vi "Begin.vi"(8 "error in":errorcluster) -> (0 "error out":errorcluster)   [LabVIEW 2014]
doc: "Called before other user functions, this VI is expected to open initial I/O refnums, load in file data, and do all program initialization. Notice that the <B>error out</B> terminal is simply used for data flow. Wiring it to other structures or subVIs ensures that this VI runs first."
uses:
  <vilib>/Rock Robotics/WPI/DriverStation/WPI_DriverStationRobotMode2.ctl
  <vilib>/Rock Robotics/WPI/Joystick/WPI_JoystickDeviceEnum.ctl
  <vilib>/Rock Robotics/SystemInterfaces/DIO/FPGA_DIOChannel.ctl
  <vilib>/Rock Robotics/SystemInterfaces/AI/FPGA_AIChannel.ctl
  <vilib>/Rock Robotics/SystemInterfaces/Typedef/FPGA_TypedefAnalogModule.ctl
  <vilib>/Rock Robotics/SystemInterfaces/DIO/FPGA_DIORelayChannel.ctl
  <vilib>/Rock Robotics/SystemInterfaces/DIO/FPGA_DIOPWMChannel.ctl
  <vilib>/Rock Robotics/SystemInterfaces/Typedef/FPGA_TypedefDigitalModule.ctl
  Robot Global Data.vi
  <vilib>/Rock Robotics/Network Tables/SD Write String Array.vi
  <vilib>/Rock Robotics/WPI/Counter/WPI_CounterDigitalInputToDigitalSource.vi
  <vilib>/Rock Robotics/WPI/MotorControl/WPI_MotorControlOpen Talon.vi
  <vilib>/Rock Robotics/WPI/Compressor/WPI_CompressorGetSetRefNum.vi
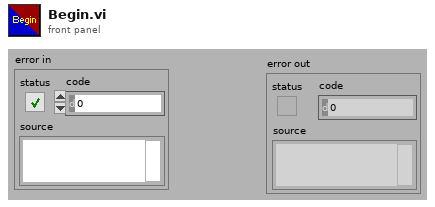
[diagram p1: front panel]
types:
  T1 = typedef "FPGA_TypedefDigitalModule.ctl" = enum16{"Controller 1"}
  T2 = typedef "FPGA_DIOPWMChannel.ctl" = enum8{"PWM 0", "PWM 1", "PWM 2", "PWM 3", "PWM 4", "PWM 5", "PWM 6", "PWM 7", "PWM 8", "PWM 9", "PWM MXP 0", "PWM MXP 1", "PWM MXP 2", "PWM MXP 3", "PWM MXP 4", "PWM MXP 5", "PWM MXP 6", "PWM MXP 7", "PWM MXP 8", "PWM MXP 9", "Invalid"}
  T3 = typedef "FPGA_DIOChannel.ctl" = enum8{"DIO 0", "DIO 1", "DIO 2", "DIO 3", "DIO 4", "DIO 5", "DIO 6", "DIO 7", "DIO 8", "DIO 9", "DIO MXP 0", "DIO MXP 1", "DIO MXP 2", "DIO MXP 3", "DIO MXP 4", "DIO MXP 5", "DIO MXP 6", "DIO MXP 7", "DIO MXP 8", "DIO MXP 9", "DIO MXP 10", "DIO MXP 11", "DIO MXP 12", "DIO MXP 13", "DIO MXP 14", "DIO MXP 15", "Invalid"}
  T4 = typedef "FPGA_DIORelayChannel.ctl" = enum8{"Relay 0", "Relay 1", "Relay 2", "Relay 3", "Invalid"}
  T5 = typedef "FPGA_TypedefAnalogModule.ctl" = enum16{"Controller 1"}
  T6 = typedef "FPGA_AIChannel.ctl" = enum8{"AI 0", "AI 1", "AI 2", "AI 3", "AI MXP 0", "AI MXP 1", "AI MXP 2", "AI MXP 3", "Invalid"}
  T7 = typedef "WPI_JoystickDeviceEnum.ctl" = enum16{"USB 0", "USB 1", "USB 2", "USB 3", "USB 4", "USB 5"}
  T8 = typedef "WPI_DriverStationRobotMode2.ctl" = enum16{"Autonomous Disabled", "Autonomous Enabled", "Teleop Disabled", "Teleop Enabled", "Disconnected", "Finish", "Test Disabled", "Test Enabled", "Emergency Stopped"}
  T9 = typedef "WPI_MotorControlDeviceRef.ctl" = cluster{"DeviceStatus":errorcluster, "Type":T10, "PWM":cluster{"Controller":T1, "PWM Channel":T2, "DeadBand":T11}, "CAN":cluster{"Device Number":u8, "Control Mode":T12, "Semaphore":T13, "Max Vout":dbl, "TalonSRX Control Mode":T14}, "Invert":bool, "TransformRef":T15, "InvTransformRef":T15}
  T10 = typedef "WPI_MotorControlType.ctl" = enum16{"PWM", "CAN", "CANTalonSRX"}
  T11 = typedef "WPI_PWMDeadband.ctl" = cluster{"Name":string, "maxPositivePwm":i32, "minPositivePwm":i32, "centerPwm":i32, "maxNegativePwm":i32, "minNegativePwm":i32, "angularRange":u16}
  T12 = typedef "WPI_CANJaguar_ControlMode.ctl" = enum8{"Percent VBus", "Current", "Speed", "Position", "Voltage"}
  T13 = typedef "Semaphore RefNum" = refnum<k1>
  T14 = typedef "WPI_CANTalonSRX_APIControlMode.ctl" = enum8{"Percent VBus", "Speed", "Position", "Slave", "Unchanged / Invalid"}
  T15 = typedef "WPI_PWMTransform_ConPane.ctl" = refnum<vi>
  T16 = typedef "WPI_DigitalInputDevRef.ctl" = cluster{"DevStatus":errorcluster, "DIO Channel":T3, "Controller":T1}
  T17 = typedef "FPGA_CounterEncoderSourceConvertionLVSourceType.ctl" = cluster{"DevStatus":errorcluster, "AnalogTriggerMode?":bool, "DigitalMode":cluster{"Controller":T1, "DIO Channel":T18}, "AnalogTriggerMode":cluster{"AnalogTriggerIndex":T19, "OutputType":T20}}
  T18 = typedef "FPGA_DIODigitalSourceChannel.ctl" = enum8{"DIO 0", "DIO 1", "DIO 2", "DIO 3", "DIO 4", "DIO 5", "DIO 6", "DIO 7", "DIO 8", "DIO 9", "DIO MXP 0", "DIO MXP 1", "DIO MXP 2", "DIO MXP 3", "DIO MXP 4", "DIO MXP 5", "DIO MXP 6", "DIO MXP 7", "DIO MXP 8", "DIO MXP 9", "DIO MXP 10", "DIO MXP 11", "DIO MXP 12", "DIO MXP 13", "DIO MXP 14", "DIO MXP 15", "Disabled"}
  T19 = typedef "FPGA_AnalogTriggerIndex.ctl" = enum8{"Trig 0", "Trig 1", "Trig 2", "Trig 3", "Trig 4", "Trig 5", "Trig 6", "Trig 7", "Invalid"}
  T20 = typedef "FPGA_AnalogTriggerOutType.ctl" = enum16{"InWindow", "TriggerState", "Rising", "Falling"}
  T21 = typedef "WPI_EncoderDevRef.ctl" = cluster{"DevStatus":errorcluster, "EncoderIndex":T22, "CounterIndex":T23, "DistancePerCount":dbl, "Decoding Type":T24}
  T22 = typedef "FPGA_EncoderIdx.ctl" = enum8{"Enc 0", "Enc 1", "Enc 2", "Enc 3", "Enc 4", "Enc 5", "Enc 6", "Enc 7", "Invalid"}
  T23 = typedef "FPGA_CounterCtrSystemIndex.ctl" = enum8{"Ctr 0", "Ctr 1", "Ctr 2", "Ctr 3", "Ctr 4", "Ctr 5", "Ctr 6", "Ctr 7", "Invalid"}
  T24 = typedef "WPI_EncoderType.ctl" = enum16{"1x", "2x", "4x"}
  T25 = typedef "WPI_RelayDevRef.ctl" = cluster{"DevStatus":errorcluster, "Relay Channel":T4, "Controller":T1, "Relay Direction":T26}
  T26 = typedef "WPI_RelayDirection.ctl" = enum16{"Both directions", "Forward only", "Reverse only"}
  T27 = typedef "WPI_CompressorDevRef.ctl" = cluster{"DevStatus":errorcluster, "Pneumatics Control Module":u8}
  T28 = typedef "WPI_JoystickDevRef.ctl" = cluster{"Device":T7}
  T29 = typedef "WPI_AnalogChannelDevRef.ctl" = cluster{"DevStatus":errorcluster, "Controller":T5, "Analog Channel":T6}
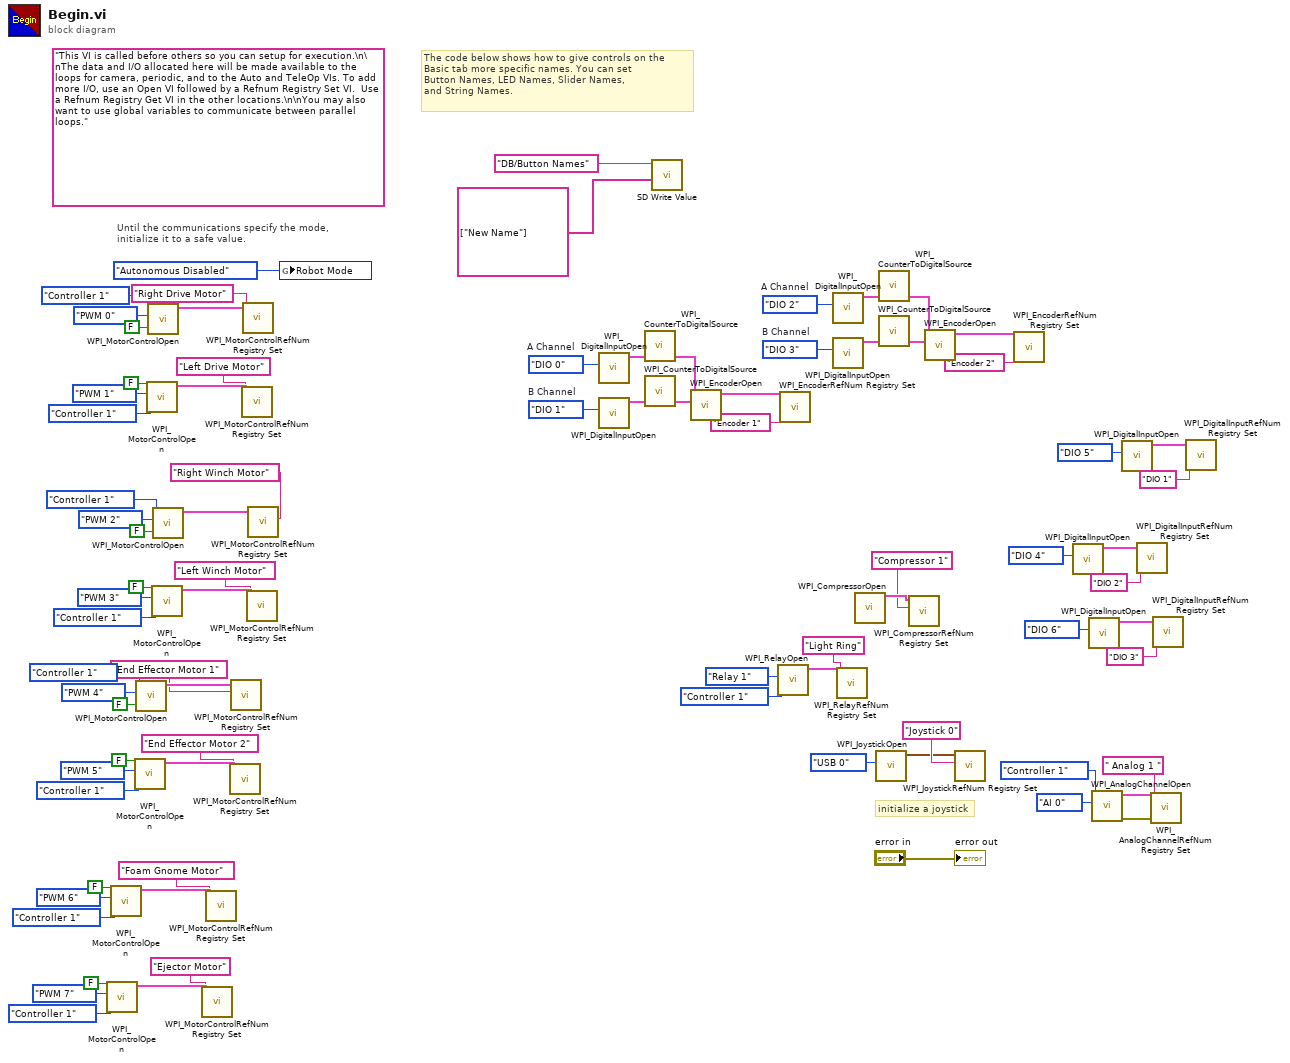
[diagram p0: block diagram]
diagram:
  w65 = FPGA_DIOChannel."DIO 3"  # B Channel
  w64 = FPGA_DIOChannel."DIO 2"  # A Channel
  w76 = FPGA_DIOChannel."DIO 1"  # B Channel
  w75 = FPGA_DIOChannel."DIO 0"  # A Channel
  (unwired) "This VI is called before others so you can setup for execution.\n\nThe data and I/O allocated here will be made available to the loops for camera, periodic, and to the Auto and TeleOp VIs. To add more I/O, use an Open VI followed by a Refnum Registry Set VI.  Use a Refnum Registry Get VI in the other locations.\n\nYou may also want to use global variables to communicate between parallel loops."
  # "The code below shows how to give controls on the\nBasic tab more specific names. You can set\nButton Names, LED Names, Slider Names,\nand String Names."
  # "initialize a joystick"
  # "Until the communications specify the mode,\ninitialize it to a safe value."
  n1 = call-poly <vilib>:"WPI_MotorControlOpen.vi"("Eliminate Deadband"=FALSE, "PWM Channel"=FPGA_DIOPWMChannel."PWM 7", "Controller"=FPGA_TypedefDigitalModule."Controller 1") -> ("MotorControlDeviceRef"=w7:T9)  [unwired: 7 in, 1 out]
  n2 = call-poly <vilib>:"WPI_MotorControlOpen.vi"("Eliminate Deadband"=FALSE, "PWM Channel"=FPGA_DIOPWMChannel."PWM 6", "Controller"=FPGA_TypedefDigitalModule."Controller 1") -> ("MotorControlDeviceRef"=w12:T9)  [unwired: 7 in, 1 out]
  n3 = call-poly <vilib>:"WPI_MotorControlOpen.vi"("Eliminate Deadband"=FALSE, "PWM Channel"=FPGA_DIOPWMChannel."PWM 5", "Controller"=FPGA_TypedefDigitalModule."Controller 1") -> ("MotorControlDeviceRef"=w20:T9)  [unwired: 7 in, 1 out]
  n4 = call-poly <vilib>:"WPI_MotorControlOpen.vi"("Eliminate Deadband"=FALSE, "PWM Channel"=FPGA_DIOPWMChannel."PWM 4", "Controller"=FPGA_TypedefDigitalModule."Controller 1") -> ("MotorControlDeviceRef"=w21:T9)  [unwired: 7 in, 1 out]
  n5 = call-poly <vilib>:"WPI_MotorControlOpen.vi"("Eliminate Deadband"=FALSE, "PWM Channel"=FPGA_DIOPWMChannel."PWM 1", "Controller"=FPGA_TypedefDigitalModule."Controller 1") -> ("MotorControlDeviceRef"=w39:T9)  [unwired: 7 in, 1 out]
  n6 = call-poly <vilib>:"WPI_MotorControlOpen.vi"("Eliminate Deadband"=FALSE, "PWM Channel"=FPGA_DIOPWMChannel."PWM 0", "Controller"=FPGA_TypedefDigitalModule."Controller 1") -> ("MotorControlDeviceRef"=w40:T9)  [unwired: 7 in, 1 out]
  n7 = call-poly <vilib>:"WPI_MotorControlOpen.vi"("Eliminate Deadband"=FALSE, "PWM Channel"=FPGA_DIOPWMChannel."PWM 3", "Controller"=FPGA_TypedefDigitalModule."Controller 1") -> ("MotorControlDeviceRef"=w29:T9)  [unwired: 7 in, 1 out]
  n8 = call-poly <vilib>:"WPI_MotorControlOpen.vi"("Eliminate Deadband"=FALSE, "PWM Channel"=FPGA_DIOPWMChannel."PWM 2", "Controller"=FPGA_TypedefDigitalModule."Controller 1") -> ("MotorControlDeviceRef"=w30:T9)  [unwired: 7 in, 1 out]
  n9 = call <vilib>:"WPI_MotorControlRefNum Registry Set.vi"("refnum name"="Ejector Motor", "MotorControlDevRef"=w7) -> ()  [unwired: 8 in, 2 out]
  n10 = call <vilib>:"WPI_MotorControlRefNum Registry Set.vi"("refnum name"="Foam Gnome Motor", "MotorControlDevRef"=w12) -> ()  [unwired: 8 in, 2 out]
  n11 = call <vilib>:"WPI_MotorControlRefNum Registry Set.vi"("refnum name"="End Effector Motor 2", "MotorControlDevRef"=w20) -> ()  [unwired: 8 in, 2 out]
  n12 = call <vilib>:"WPI_MotorControlRefNum Registry Set.vi"("refnum name"="End Effector Motor 1", "MotorControlDevRef"=w21) -> ()  [unwired: 8 in, 2 out]
  n13 = call <vilib>:"WPI_MotorControlRefNum Registry Set.vi"("refnum name"="Left Drive Motor", "MotorControlDevRef"=w39) -> ()  [unwired: 8 in, 2 out]
  n14 = call <vilib>:"WPI_MotorControlRefNum Registry Set.vi"("refnum name"="Right Drive Motor", "MotorControlDevRef"=w40) -> ()  [unwired: 8 in, 2 out]
  n15 = call <vilib>:"WPI_MotorControlRefNum Registry Set.vi"("refnum name"="Left Winch Motor", "MotorControlDevRef"=w29) -> ()  [unwired: 8 in, 2 out]
  n16 = call <vilib>:"WPI_MotorControlRefNum Registry Set.vi"("refnum name"="Right Winch Motor", "MotorControlDevRef"=w30) -> ()  [unwired: 8 in, 2 out]
  n17 = global write "Robot Global Data.vi" "Robot Mode"(WPI_DriverStationRobotMode2."Autonomous Disabled" ("Robot Mode")) -> ()
  n18 = call <vilib>:"WPI_DigitalInputOpen.vi"("DIO Channel"=w75) -> ("DigitalInputDevRef"=w72:T16)  [unwired: 2 in, 8 out]
  n19 = call <vilib>:"WPI_DigitalInputOpen.vi"("DIO Channel"=w76) -> ("DigitalInputDevRef"=w73:T16)  [unwired: 2 in, 8 out]
  n20 = call-poly <vilib>:"WPI_CounterToDigitalSource.vi"("DigitalInputDevRef"=w72) -> ("Digital Source"=w71:T17)  [unwired: 6 out]
  n21 = call-poly <vilib>:"WPI_CounterToDigitalSource.vi"("DigitalInputDevRef"=w73) -> ("Digital Source"=w74:T17)  [unwired: 6 out]
  n22 = call-poly <vilib>:"SD Write Value.vi"("String Array"=string[] ["New Name"], "Name"="DB/Button Names") -> ()  [unwired: 8 in, 2 out]
  n23 = call <vilib>:"WPI_EncoderOpen.vi"("BSource"=w74, "ASource"=w71) -> ("EncoderDevRef"=w70:T21)  [unwired: 6 in, 3 out]
  n24 = call <vilib>:"WPI_RelayOpen.vi"("Relay Channel"=FPGA_DIORelayChannel."Relay 1", "Controller"=FPGA_TypedefDigitalModule."Controller 1") -> ("RelayDevRef"=w50:T25)  [unwired: 8 in, 1 out]
  n25 = call <vilib>:"WPI_EncoderRefNum Registry Set.vi"("refnum name"="Encoder 1", "EncoderDevRef"=w70) -> ()  [unwired: 8 in, 2 out]
  n26 = call <vilib>:"WPI_DigitalInputOpen.vi"("DIO Channel"=w64) -> ("DigitalInputDevRef"=w61:T16)  [unwired: 2 in, 8 out]
  n27 = call <vilib>:"WPI_DigitalInputOpen.vi"("DIO Channel"=w65) -> ("DigitalInputDevRef"=w62:T16)  [unwired: 2 in, 8 out]
  n28 = call <vilib>:"WPI_RelayRefNum Registry Set.vi"("refnum name"="Light Ring", "RelayDevRef"=w50) -> ()  [unwired: 8 in, 2 out]
  n29 = call <vilib>:"WPI_CompressorOpen.vi"() -> ("CompressorDevRef"=w57:T27)  [unwired: 14 in, 1 out]
  n30 = call <vilib>:"WPI_JoystickOpen.vi"("JoystickDevice"=WPI_JoystickDeviceEnum."USB 0") -> ("JoystickDevRef"=w81:T28)  [unwired: 10 in]
  n31 = call-poly <vilib>:"WPI_CounterToDigitalSource.vi"("DigitalInputDevRef"=w61) -> ("Digital Source"=w60:T17)  [unwired: 6 out]
  n32 = call-poly <vilib>:"WPI_CounterToDigitalSource.vi"("DigitalInputDevRef"=w62) -> ("Digital Source"=w63:T17)  [unwired: 6 out]
  n33 = call <vilib>:"WPI_CompressorRefNum Registry Set.vi"("refnum name"="Compressor 1", "CompressorDevRef"=w57) -> ()  [unwired: 8 in, 2 out]
  n34 = call <vilib>:"WPI_EncoderOpen.vi"("BSource"=w63, "ASource"=w60) -> ("EncoderDevRef"=w59:T21)  [unwired: 6 in, 3 out]
  n35 = call <vilib>:"WPI_JoystickRefNum Registry Set.vi"("refnum name"="Joystick 0", "JoystickDevRef"=w81) -> ()  [unwired: 8 in, 2 out]
  n36 = call <vilib>:"WPI_EncoderRefNum Registry Set.vi"("refnum name"="Encoder 2", "EncoderDevRef"=w59) -> ()  [unwired: 8 in, 2 out]
  n37 = call <vilib>:"WPI_DigitalInputOpen.vi"("DIO Channel"=FPGA_DIOChannel."DIO 4") -> ("DigitalInputDevRef"=w42:T16)  [unwired: 9 in, 1 out]
  n38 = call <vilib>:"WPI_DigitalInputOpen.vi"("DIO Channel"=FPGA_DIOChannel."DIO 6") -> ("DigitalInputDevRef"=w67:T16)  [unwired: 9 in, 1 out]
  n39 = call <vilib>:"WPI_AnalogChannelOpen.vi"("Analog Channel"=FPGA_AIChannel."AI 0", "Controller"=FPGA_TypedefAnalogModule."Controller 1") -> ("error out"=w55:errorcluster, "AIDeviceRef"=w54:T29)  [unwired: 8 in]
  n40 = call <vilib>:"WPI_DigitalInputOpen.vi"("DIO Channel"=FPGA_DIOChannel."DIO 5") -> ("DigitalInputDevRef"=w45:T16)  [unwired: 9 in, 1 out]
  n41 = call <vilib>:"WPI_DigitalInputRefNum Registry Set.vi"("refnum name"="DIO 2", "DigitalInputDevRef"=w42) -> ()  [unwired: 8 in, 2 out]
  n42 = call <vilib>:"WPI_AnalogChannelRefNum Registry Set.vi"("error in (no error)"=w55, "refnum name"=" Analog 1 ", "AIDeviceRef"=w54) -> ()  [unwired: 7 in, 2 out]
  n43 = call <vilib>:"WPI_DigitalInputRefNum Registry Set.vi"("refnum name"="DIO 3", "DigitalInputDevRef"=w67) -> ()  [unwired: 8 in, 2 out]
  n44 = call <vilib>:"WPI_DigitalInputRefNum Registry Set.vi"("refnum name"="DIO 1", "DigitalInputDevRef"=w45) -> ()  [unwired: 8 in, 2 out]
  "error out" <- "error in"
